vi "Shared_Initialize.vi"(9 "Simulated HW?":bool, 10 "Driver":T1(ring), 11 "Semiconductor Module Context":T2) -> (0 "error out":errorcluster)   [LabVIEW 2023, in "Shared.lvlib"]
doc: "Initializes driver sessions, DCPower, PPMU, FGEN, SCOPE, Relay Driver"
uses:
  Shared.lvlib
  <vilib>/NI_TestStand_SemiconductorModule/NI_TestStand_Semiconductor_Module.lvlibp/PinMap/General/SemiconductorModuleContext.ctl
  <vilib>/NI_TestStand_SemiconductorModule/NI_TestStand_Semiconductor_Module.lvlibp
  ResourceHandling/ResourceHandling.lvlib
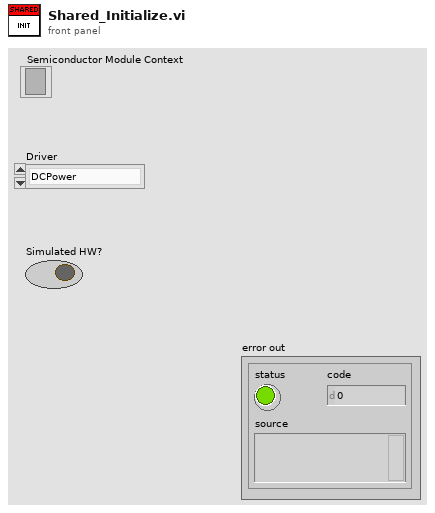
[diagram p1: front panel]
types:
  T1 = enum16{"DCPower", "SCOPE", "FGEN", "Relays", "PPMU"}
  T2 = typedef "NI_TestStand_Semiconductor_Module.lvlibp/SemiconductorModuleContext.ctl" = refnum<k7>
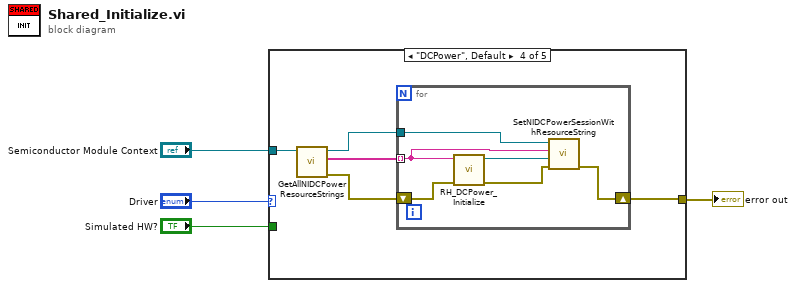
[diagram p0: block diagram]
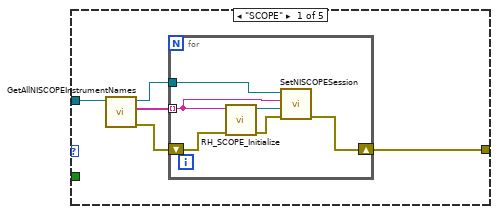
[diagram p2: hidden frame]
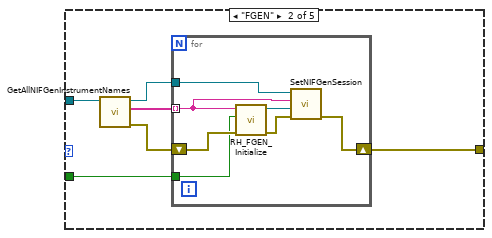
[diagram p3: hidden frame]
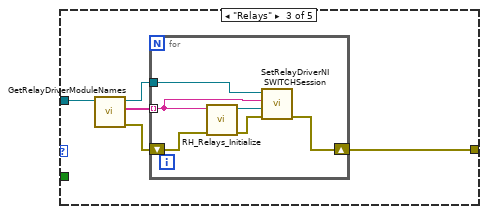
[diagram p4: hidden frame]
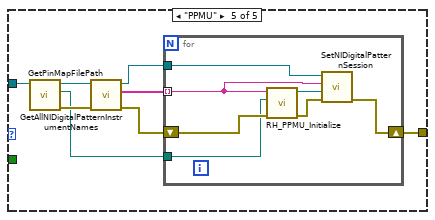
[diagram p5: hidden frame]
diagram:
  n1 = case shown="\"DCPower\", Default" "Driver" {
    tunnel: "Semiconductor Module Context" -> [w9 w21 w33 w43 w53]
    tunnel: [w5 w17 w29 w44 w55] -> w3
    tunnel: "Simulated HW?" -> [_ w16 _ _ _]
    frame "SCOPE" {
      n2 = call <vilib>:"GetAllNISCOPEInstrumentNames.vi"("Semiconductor Module Context"=w9) -> ("error out"=w7:errorcluster, "Instrument Names"=w6:string[], "Semiconductor Module Context Out"=w8:T2)  [unwired: 8 in]
      n3 = for {
        tunnel: w8 -> [w14]
        tunnel: w6 -> [w13] mode=indexing
        shift-right: [w11] -> w5
        shift-left: w7 -> [w15]
        n4 = call "RH_SCOPE_Initialize.vi"("error in"=w15, "SCOPE Resource Name"=w13) -> ("error out"=w12:errorcluster, "SCOPE Session Out"=w10:refnum<k15>)  [unwired: 8 in]
        n5 = call <vilib>:"SetNISCOPESession.vi"("error in (no error)"=w12, "Instrument Session"=w10, "Instrument Name"=w13, "Semiconductor Module Context"=w14) -> ("error out"=w11:errorcluster)  [unwired: 6 in, 1 out]
      }
    }
    frame "FGEN" {
      n6 = call <vilib>:"GetAllNIFGenInstrumentNames.vi"("Semiconductor Module Context"=w21) -> ("error out"=w19:errorcluster, "Instrument Names"=w18:string[], "Semiconductor Module Context Out"=w20:T2)  [unwired: 8 in]
      n7 = for {
        tunnel: w20 -> [w27]
        tunnel: w18 -> [w25] mode=indexing
        shift-right: [w23] -> w17
        shift-left: w19 -> [w28]
        tunnel: w16 -> [w22]
        n8 = call "RH_FGEN_Initialize.vi"("error in"=w28, "Simulated HW?"=w22, "Resource Name"=w25) -> ("error out"=w24:errorcluster, "FGEN Session Out"=w26:refnum<k15>)  [unwired: 7 in]
        n9 = call <vilib>:"SetNIFGenSession.vi"("error in (no error)"=w24, "Instrument Session"=w26, "Instrument Name"=w25, "Semiconductor Module Context"=w27) -> ("error out"=w23:errorcluster)  [unwired: 6 in, 1 out]
      }
    }
    frame "Relays" {
      n10 = call <vilib>:"GetRelayDriverModuleNames.vi"("Semiconductor Module Context"=w33) -> ("error out"=w31:errorcluster, "Module Names"=w30:string[], "Semiconductor Module Context Out"=w32:T2)  [unwired: 8 in]
      n11 = for {
        tunnel: w32 -> [w38]
        tunnel: w30 -> [w36] mode=indexing
        shift-right: [w34] -> w29
        shift-left: w31 -> [w39]
        n12 = call "RH_Relays_Initialize.vi"("error in"=w39, "Relays Resource Name"=w36) -> ("error out"=w35:errorcluster, "Relays Session Out"=w37:refnum<k15>)  [unwired: 8 in]
        n13 = call <vilib>:"SetRelayDriverNISWITCHSession.vi"("error in (no error)"=w35, "NI-SWITCH Session"=w37, "Relay Driver Module Name"=w36, "Semiconductor Module Context"=w38) -> ("error out"=w34:errorcluster)  [unwired: 6 in, 1 out]
      }
    }
    frame "DCPower", Default {
      n14 = call <vilib>:"GetAllNIDCPowerResourceStrings.vi"("Semiconductor Module Context"=w43) -> ("error out"=w41:errorcluster, "Resource Strings"=w40:string[], "Semiconductor Module Context Out"=w42:T2)  [unwired: 8 in]
      n15 = for {
        tunnel: w42 -> [w49]
        tunnel: w40 -> [w45] mode=indexing
        shift-right: [w47] -> w44
        shift-left: w41 -> [w50]
        n16 = call "RH_DCPower_Initialize.vi"("error in"=w50, "resource name"=w45) -> ("error out"=w48:errorcluster, "DCPower Session Out"=w46:refnum<k15>)  [unwired: 8 in]
        n17 = call <vilib>:"SetNIDCPowerSessionWithResourceString.vi"("error in (no error)"=w48, "Instrument Session"=w46, "Resource String"=w45, "Semiconductor Module Context"=w49) -> ("error out"=w47:errorcluster)  [unwired: 6 in, 1 out]
      }
    }
    frame "PPMU" {
      n18 = call <vilib>:"GetPinMapFilePath.vi"("Semiconductor Module Context"=w53) -> ("error out"=w52:errorcluster, "Pin Map File Path"=w51:path, "Semiconductor Module Context Out"=w54:T2)  [unwired: 8 in]
      n19 = call <vilib>:"GetAllNIDigitalPatternInstrumentNames.vi"("error in (no error)"=w52, "Semiconductor Module Context"=w54) -> ("error out"=w57:errorcluster, "Instrument Names"=w56:string[], "Semiconductor Module Context Out"=w58:T2)  [unwired: 7 in]
      n20 = for {
        tunnel: w58 -> [w64]
        tunnel: w56 -> [w62] mode=indexing
        shift-right: [w60] -> w55
        shift-left: w57 -> [w65]
        tunnel: w51 -> [w59]
        n21 = call "RH_PPMU_Initialize.vi"("error in"=w65, "pin map file"=w59, "PPMU Resource Name"=w62) -> ("error out"=w61:errorcluster, "PPMU Session Out"=w63:refnum<k15>)  [unwired: 6 in]
        n22 = call <vilib>:"SetNIDigitalPatternSession.vi"("error in (no error)"=w61, "Instrument Session"=w63, "Instrument Name"=w62, "Semiconductor Module Context"=w64) -> ("error out"=w60:errorcluster)  [unwired: 6 in, 1 out]
      }
    }
  }
  "error out" <- w3
